vi "S2C_LoopCount.vi"(8 "Error In":errorcluster, 11 "MenuRef":refnum<k9>) -> (0 "Error Out":errorcluster)   [LabVIEW 2015]
doc: "Toggles the \"Local File\" runtime menu item."
uses:
  Globals/S2C_Globals.vi
panel:
  out "Init":bool
  in  "Done":bool
  in  "Loops":i32 caption="Number of Loops" min=-1 step=1
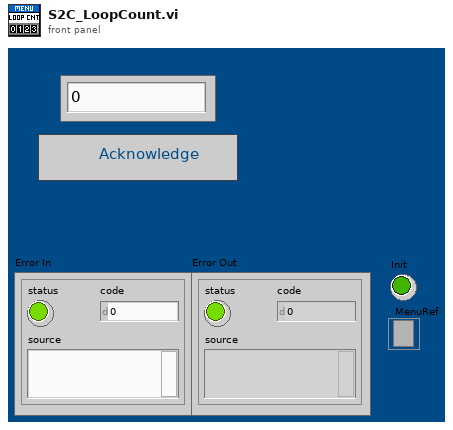
[diagram p1: front panel]
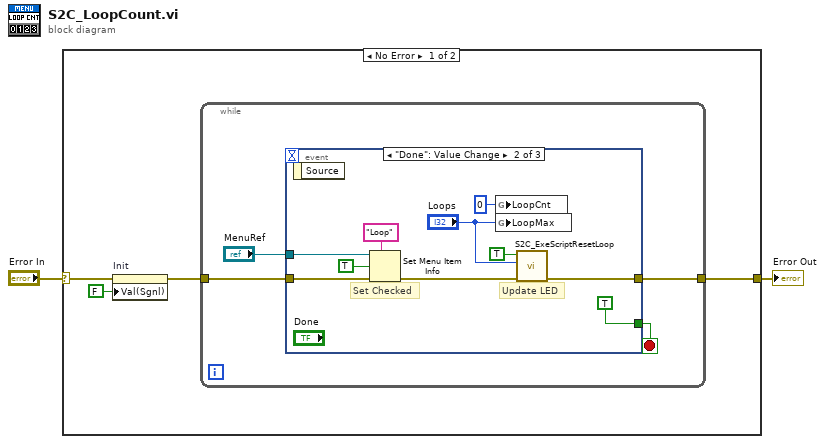
[diagram p0: block diagram]
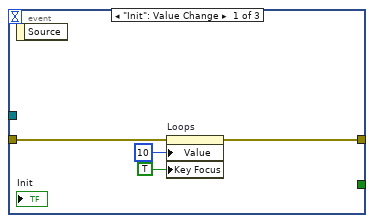
[diagram p2: hidden frame]
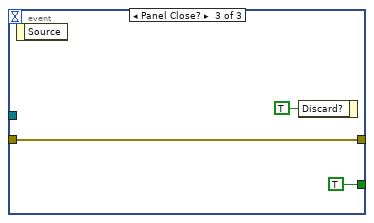
[diagram p3: hidden frame]
diagram:
  n1 = case shown="No Error" "Error In" {
    selector: "Error In" -> [w5 w28]
    tunnel: [w6 w28] -> w1
    frame No Error {
      n2 = property on="Init" class="Bool (strict)"(error in=w5, "Val(Sgnl)"=FALSE ("Value (Signaling)")) -> (error out=w4:errorcluster)  [unwired: 1 in, 1 out]
      n3 = while {
        tunnel: w4 -> [w10]
        tunnel: [w9] -> w6
        stop <- w8 stop-if-true
        n4 = event shown="[1] \"Done\": Value Change" {
          selector: _ -> [_ _ _]
          dyn-events: _ -> [_ _ _]
          timeout: _ -> [_ _ _]
          tunnel: w10 -> [w14 w20 w25]
          tunnel: [w13 w21 w25] -> w9
          tunnel: [_ TRUE TRUE] -> w8
          tunnel: "MenuRef" -> [_ w19 _]
          event "Init": Value Change {
            n5 = event-data() -> ()  [unwired: 1 in, 1 out]
            n6 = property on="Loops" class="DigNum (strict)"(error in=w14, "Value"=10 ("Loops"), "Key Focus"=TRUE) -> (error out=w13:errorcluster)  [unwired: 1 in, 1 out]
          }
          event "Done": Value Change {
            # "Set Checked"
            # "Update LED"
            n7 = event-data() -> ()  [unwired: 1 in, 1 out]
            n8 = Set Menu Item Info(6:TRUE ("checked"), 7:"Loop" ("item tag"), 8:w20, 11:w19) -> (0:w16:errorcluster)  [unwired: 3 in, 1 out]
            n9 = global write "S2C_Globals.vi" "LoopCnt"(0 ("LoopCnt")) -> ()
            n10 = global write "S2C_Globals.vi" "LoopMax"("Loops") -> ()
            n11 = call "S2C_ExeScriptResetLoop.vi"("Error In"=w16, "Loops"="Loops", "Loop?"=TRUE) -> ("Error Out"=w21:errorcluster)  [unwired: 8 in]
          }
          event Panel Close? {
            n12 = event-data() -> ()  [unwired: 1 in, 1 out]
            n13 = event-data("Discard?"=TRUE) -> ()  [unwired: 1 in, 1 out]
          }
        }
      }
    }
    frame Error {
    }
  }
  "Error Out" <- w1
